vi "Remove Comments from Line.vi"(3 "Single-line Text":string) -> (1 "Single-line Text Without Comments":string)   [LabVIEW 2017, in "Communicable State Machine.lvlib"]
doc: "-- <b>Controls</b> --\n- <b>single-line text</b>:\n\n-- <b>Indicators</b> --\n- <b>single-line text without comments</b>:"
uses:
  Communicable State Machine.lvlib
  _Shared/CSM Shared.lvlib
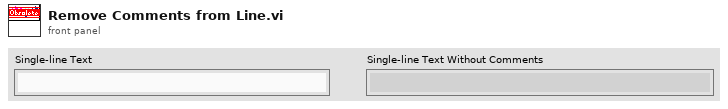
[diagram p1: front panel]
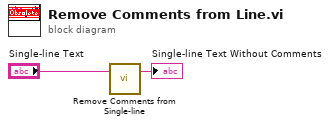
[diagram p0: block diagram]
diagram:
  n1 = call "Remove Comments from Single-line.vi"("single-line text"="Single-line Text") -> ("single-line text without comments"=→"Single-line Text Without Comments":string)  [unwired: 2 in]
